vi "Get CallerWatchdog Queue.vi"(8 "error in (no error)":errorcluster, 11 "SMO in":refnum<class "SMO.lvclass">) -> (0 "error out":errorcluster, 2 "Caller Watchdog":refnum<queue>, 3 "SMO out":refnum<class "SMO.lvclass">)   [LabVIEW 2021, in "smo.lvlib" / "SMO.lvclass"]
uses:
  SMO.lvclass
  SMO.lvclass/SMO.ctl
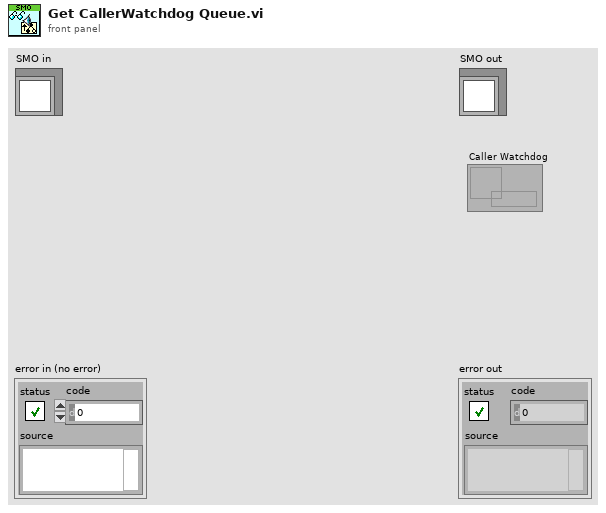
[diagram p1: front panel]
types:
  T1 = typedef "smo.lvlib/SMO.lvclass/PrivateData--Ref.ctl" = refnum<data-value>
  T2 = typedef "smo.lvlib/SMO.lvclass/PrivateData--Cluster.ctl" = cluster{"Parent Call":T3, "Registered Processes":T4[], "Sync Notifier":refnum<notifier>, "Process Error Notifier":refnum<notifier>, "Protected Events":T5, "Public Events":T6, "SMO State":T7, "[Attributes]":variant, "Launcher Close":refnum<notifier>, "Caller Watchdog":refnum<queue>, "Accessibility":T8, "NbStaticDependencies":u32}
  T3 = typedef "smo.lvlib/SMO.lvclass/Parent Call--Enum.ctl" = enum16{"Allows parent to run", "Does not request parent to run"}
  T4 = typedef "smo.lvlib/SMO.lvclass/RegisteredProcessData--Cluster.ctl" = cluster{"Name":string, "Static VI Ref":refnum<vi>, "Running":bool, "NotifierRef":u32}
  T5 = typedef "smo.lvlib/SMO.lvclass/Protected Events.ctl" = cluster{"StopProcesses":refnum<user-event>, "AbortProcesses":refnum<user-event>, "Config Changed":refnum<user-event>, "Dependency":refnum<user-event>}
  T6 = typedef "smo.lvlib/SMO.lvclass/Public Events.ctl" = cluster{"Error":refnum<user-event>, "State":refnum<user-event>, "Reserve State":refnum<user-event>}
  T7 = typedef "smo.lvlib/SMO.lvclass/SMOState --Enum.ctl" = enum16{"unknown", "Created", "Started", "Stopped"}
  T8 = typedef "smo.lvlib/SMO.lvclass/Accessibility--Cluster.ctl" = cluster{"Lock Key":string, "Reserve State":T9}
  T9 = typedef "smo.lvlib/SMO.lvclass/Reserve State--Enum.ctl" = enum16{"Unreserved", "Reserved", "Self-locked"}
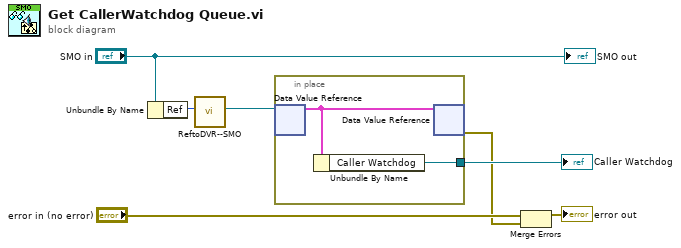
[diagram p0: block diagram]
diagram:
  n1 = Unbundle By Name("SMO in") -> ("Ref"=w4:u32)
  n2 = call "ReftoDVR--SMO.vi"("Ref"=w4) -> ("Ref"=w3:T1)  [unwired: 10 in]
  n3 = in-place {
    in-place-border: [w8] -> w5
    n4 = in-place-dvr #1(w3) -> (w9:T2)  [unwired: 1 out]
    n5 = Unbundle By Name(w9) -> ("Caller Watchdog"=w8:refnum<queue>)
    n6 = in-place-dvr #1(w9) -> (w2:errorcluster)  [unwired: 1 out]
  }
  "Caller Watchdog" <- w5
  n7 = Merge Errors("error in (no error)", w2) -> (→"error out":errorcluster)
  "SMO out" <- "SMO in"
